vi "Add Parameters.vi"(8 "error in (no error)":errorcluster, 10 "Parameters":refnum<class "Analyze Parameter Base.lvclass">[](array[class]), 11 "Analyze BaseClass in":refnum<class "Analyze BaseClass.lvclass">) -> (0 "error out":errorcluster, 3 "Analyze BaseClass out":refnum<class "Analyze BaseClass.lvclass">)   [LabVIEW 2020, in "Analyze.lvlib" / "Analyze BaseClass.lvlib" / "Analyze BaseClass.lvclass"]
uses:
  Analyze BaseClass.lvclass
  Analyze Parameter/Analyze Parameter Base/Analyze Parameter Base.lvclass
  Analyze BaseClass.lvclass/Analyze BaseClass.ctl
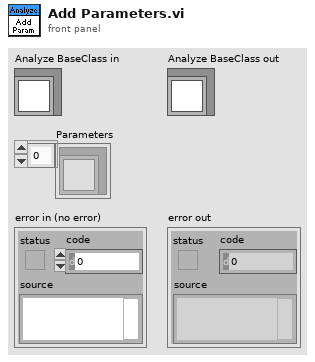
[diagram p1: front panel]
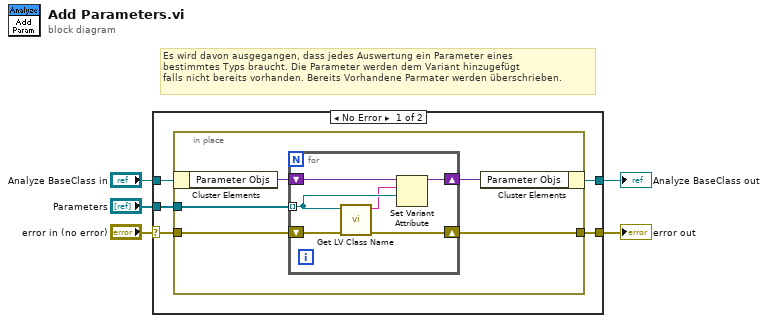
[diagram p0: block diagram]
diagram:
  # "Es wird davon ausgegangen, dass jedes Auswertung ein Parameter eines \nbestimmtes Typs braucht. Die Parameter werden dem Variant hinzugefügt\nfalls nicht bereits vorhanden. Bereits Vorhandene Parmater werden überschrieben."
  n1 = case shown="No Error" "error in (no error)" {
    selector: "error in (no error)" -> [w7 w23]
    tunnel: [w6 w23] -> w4
    tunnel: [w9 w22] -> w2
    tunnel: "Analyze BaseClass in" -> [w10 w22]
    tunnel: "Parameters" -> [w8 _]
    frame No Error {
      n2 = in-place {
        in-place-border: w8 -> [w13]
        in-place-border: w7 -> [w12]
        in-place-border: [w11] -> w6
        n3 = in-place-cluster #1(w10) -> ("Parameter Objs"=w15:variant)
        n4 = for {
          shift-right: [w20] -> w14
          shift-left: w15 -> [w21]
          tunnel: w13 -> [w19] mode=indexing
          shift-right: [w16] -> w11
          shift-left: w12 -> [w17]
          n5 = call <vilib>:"Get LV Class Name.vi"("error in (no error)"=w17, "object"=w19) -> ("error out"=w16:errorcluster, "class name"=w18:string)  [unwired: 8 in]
          n6 = Set Variant Attribute(Variant=w21, name=w18, value=w19) -> (Variant out=w20:variant)  [unwired: 1 in, 2 out]
        }
        n7 = in-place-cluster #1("Parameter Objs"=w14) -> (w9:refnum<class "Analyze BaseClass.lvclass">)
      }
    }
    frame Error {
    }
  }
  "error out" <- w4
  "Analyze BaseClass out" <- w2
